vi "Util_ConvertArrayOfStringsToString.vi"(1 "Array<string>":string[](array[string])) -> (0 "String":string)   [LabVIEW 2020]
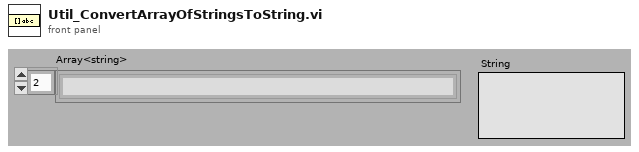
[diagram p1: front panel]
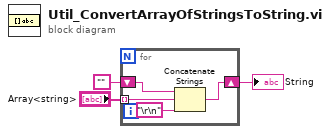
[diagram p0: block diagram]
diagram:
  n1 = for {
    tunnel: "Array<string>" -> [w7] mode=indexing
    shift-right: [w6] -> w1
    shift-left: "" -> [w5]
    n2 = Concatenate Strings(w5, w7, "\r\n") -> (w6:string)
  }
  "String" <- w1
